vi "Check Point to Point Distance.vi"(6 "fit radius":dbl, 8 "scaling info":T1={"pixels per unit"=1.0, "fit radius (units)"=1.0, "center point (pixels)"={"x"=0, "y"=0}}, 9 "max dist squared":dbl, 10 "P2 (units)":cluster{"x":dbl, "y":dbl}, 11 "P1 (units)":cluster{"x":dbl, "y":dbl}) -> (1 "valid?":bool, 2 "P2 (pixels)":cluster{"x":i16, "y":i16}, 3 "P1 (pixels)":cluster{"x":i16, "y":i16})   [LabVIEW 2017, in "NI_Robotics_2D Rangefinder Picture.lvlib"]
uses:
  <vilib>/robotics/Controls/2D Rangefinder/2D Rangefinder Picture/NI_Robotics_2D Rangefinder Picture.lvlib
  <vilib>/robotics/Controls/2D Rangefinder/2D Rangefinder Picture/Scaling Info.ctl
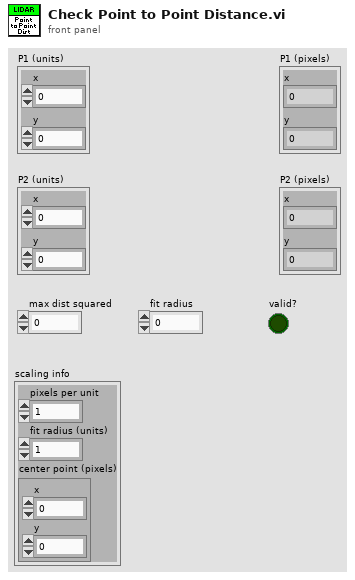
[diagram p1: front panel]
types:
  T1 = typedef "NI_Robotics_2D Rangefinder Picture.lvlib/Scaling Info.ctl" = cluster{"pixels per unit":dbl, "fit radius (units)":dbl, "center point (pixels)":cluster{"x":i16, "y":i16}}
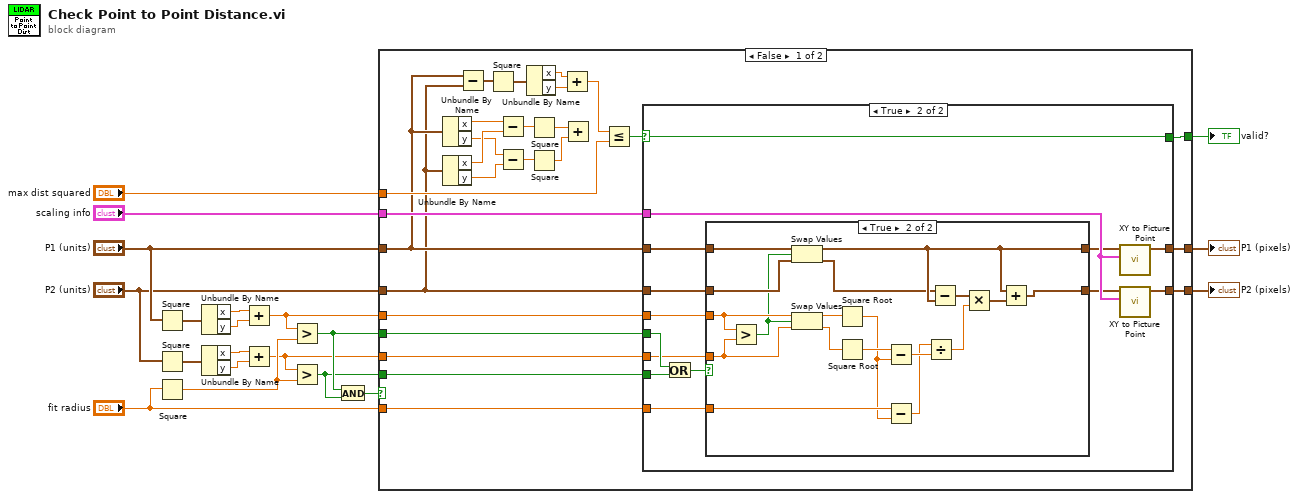
[diagram p0: block diagram]
diagram:
  n1 = Square(x="P1 (units)") -> (x^2=w9:cluster{"x":dbl, "y":dbl})
  n2 = Square(x="P2 (units)") -> (x^2=w10:cluster{"x":dbl, "y":dbl})
  n3 = Square(x="fit radius") -> (x^2=w7:dbl)
  n4 = Unbundle By Name(w9) -> ("x"=w14:dbl, "y"=w13:dbl)
  n5 = Unbundle By Name(w10) -> ("x"=w11:dbl, "y"=w12:dbl)
  n6 = Add(x=w14, y=w13) -> (x+y=w3:dbl)
  n7 = Add(x=w11, y=w12) -> (x+y=w2:dbl)
  n8 = Greater?(x=w3, y=w7) -> (0:w5:bool)
  n9 = Greater?(x=w2, y=w7) -> (0:w4:bool)
  n10 = And(x=w5, y=w4) -> (x .and. y?=w6:bool)
  n11 = case shown="False" w6 {
    tunnel: "max dist squared" -> [w38 _]
    tunnel: [w33 _] -> w19
    tunnel: "scaling info" -> [w36 _]
    tunnel: [w35 _] -> w17
    tunnel: [w34 _] -> w16
    tunnel: "P1 (units)" -> [w27 _]
    tunnel: "P2 (units)" -> [w26 _]
    tunnel: w5 -> [w32 _]
    tunnel: w4 -> [w31 _]
    tunnel: w3 -> [w30 _]
    tunnel: w2 -> [w29 _]
    tunnel: "fit radius" -> [w28 _]
    frame False {
      n12 = Unbundle By Name(w27) -> ("x"=w46:dbl, "y"=w44:dbl)
      n13 = Unbundle By Name(w26) -> ("x"=w45:dbl, "y"=w43:dbl)
      n14 = Subtract(x=w27, y=w26) -> (x-y=w25:cluster{"x":dbl, "y":dbl})
      n15 = Square(x=w25) -> (x^2=w24:cluster{"x":dbl, "y":dbl})
      n16 = Subtract(x=w46, y=w45) -> (x-y=w42:dbl)
      n17 = Subtract(x=w44, y=w43) -> (x-y=w41:dbl)
      n18 = Unbundle By Name(w24) -> ("x"=w22:dbl, "y"=w23:dbl)
      n19 = Square(x=w42) -> (x^2=w40:dbl)
      n20 = Square(x=w41) -> (x^2=w39:dbl)
      n21 = Add(x=w22, y=w23) -> (x+y=w21:dbl)
      n22 = Add(x=w40, y=w39) -> ()  [unwired: 1 out]
      n23 = Less Or Equal?(x=w21, y=w38) -> (x <= y?=w37:bool)
      n24 = case shown="True" w37 {
        selector: w37 -> [_ w57]
        tunnel: w27 -> [_ w53]
        tunnel: w26 -> [_ w51]
        tunnel: w36 -> [_ w60]
        tunnel: [_ w59] -> w35
        tunnel: [_ w58] -> w34
        tunnel: [_ w57] -> w33
        tunnel: w32 -> [_ w56]
        tunnel: w31 -> [_ w55]
        tunnel: w30 -> [_ w49]
        tunnel: w29 -> [_ w48]
        tunnel: w28 -> [_ w47]
        frame False {
        }
        frame True {
          n25 = Or(x=w56, y=w55) -> (x .or. y?=w54:bool)
          n26 = case shown="True" w54 {
            tunnel: w53 -> [w62 w80]
            tunnel: [w62 w65] -> w52
            tunnel: w51 -> [w61 w79]
            tunnel: [w61 w63] -> w50
            tunnel: w49 -> [_ w78]
            tunnel: w48 -> [_ w76]
            tunnel: w47 -> [_ w73]
            frame False {
            }
            frame True {
              n27 = Greater?(x=w78, y=w76) -> (0:w77:bool)
              n28 = Swap Values(12:w80, 13:w77, 14:w79) -> (1:w65:cluster{"x":dbl, "y":dbl}, 3:w64:cluster{"x":dbl, "y":dbl})
              n29 = Swap Values(12:w78, 13:w77, 14:w76) -> (1:w75:dbl, 3:w74:dbl)
              n30 = Square Root(x=w75) -> (sqrt(x)=w71:dbl)
              n31 = Square Root(x=w74) -> (sqrt(x)=w72:dbl)
              n32 = Subtract(x=w72, y=w71) -> (x-y=w70:dbl)
              n33 = Subtract(x=w73, y=w71) -> (x-y=w69:dbl)
              n34 = Divide(x=w69, y=w70) -> (x/y=w68:dbl)
              n35 = Subtract(x=w64, y=w65) -> (x-y=w67:cluster{"x":dbl, "y":dbl})
              n36 = Multiply(x=w67, y=w68) -> (x*y=w66:cluster{"x":dbl, "y":dbl})
              n37 = Add(x=w65, y=w66) -> (x+y=w63:cluster{"x":dbl, "y":dbl})
            }
          }
          n38 = call <vilib>:"XY to Picture Point.vi"("scaling info"=w60, "xy point (units)"=w52) -> ("xy point (pixels)"=w59:cluster{"x":i16, "y":i16})  [unwired: 9 in]
          n39 = call <vilib>:"XY to Picture Point.vi"("scaling info"=w60, "xy point (units)"=w50) -> ("xy point (pixels)"=w58:cluster{"x":i16, "y":i16})  [unwired: 9 in]
        }
      }
    }
    frame True {
      # "Both points are outside the fit radius."
    }
  }
  "valid?" <- w19
  "P1 (pixels)" <- w17
  "P2 (pixels)" <- w16
